vi "Test Shift Registers Loop 1.vi"() -> ()   [LabVIEW 2014]
panel:
  out "Array":string[](array[string])
  out "elements class name and label 2":string[](array[string])
  out "elements class name and label":string[](array[string])
  in  "vi path":path=path "C:/Users/lubo/Documents/LabView/LabVIEW-Universal-Transcriptor/Test/Examples For Parsing/Example System Functions.vi"
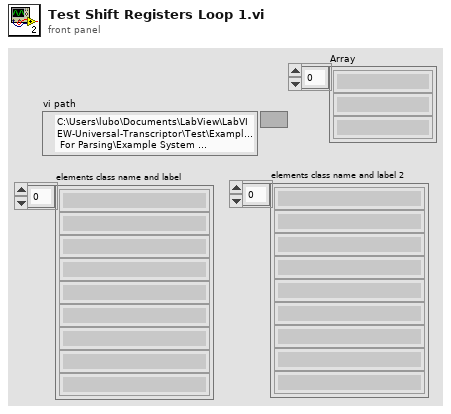
[diagram p1: front panel]
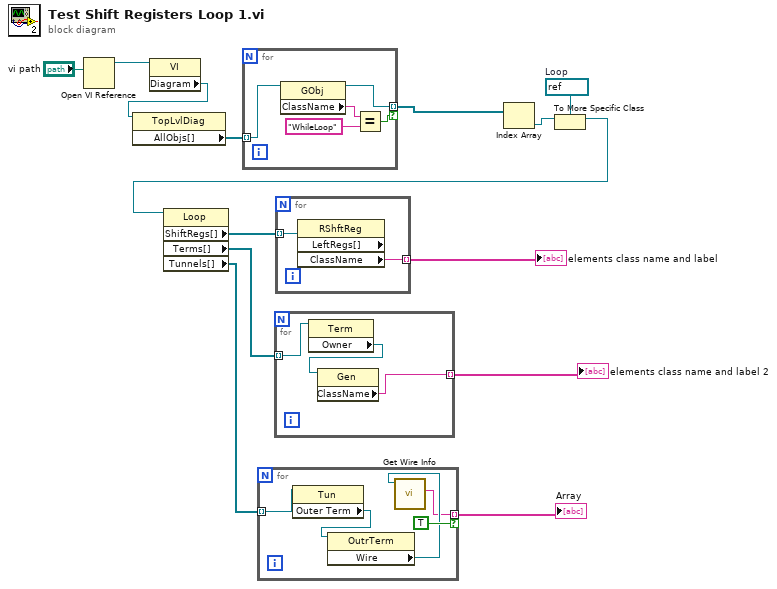
[diagram p0: block diagram]
diagram:
  w8 = refnum<vi> refnum  # Loop
  n1 = Open VI Reference(vi path="vi path") -> (vi reference=w13:refnum<vi>)  [unwired: 5 in, 1 out]
  n2 = property class="VI"(reference=w13) -> ("Diagram"=w12:refnum<vi>)  [unwired: 1 in, 2 out]
  n3 = property class="TopLvlDiag"(reference=w12) -> ("AllObjs[]"=w11:refnum<vi>[])  [unwired: 1 in, 2 out]
  n4 = for {
    tunnel: w11 -> [w19] mode=indexing
    tunnel: [w17] -> w10 mode=indexing if=w18
    n5 = property class="GObj"(reference=w19) -> (reference out=w17:refnum<vi>, "ClassName"=w15:string)  [unwired: 1 in, 1 out]
    n6 = Equal?(x=w15, y="WhileLoop") -> (x = y?=w18:bool)
  }
  n7 = Index Array(array=w10) -> (element=w9:refnum<vi>)  [unwired: 1 in]
  n8 = To More Specific Class(target class=w8, reference=w9) -> (specific class reference=w7:refnum<vi>)  [unwired: 1 in, 1 out]
  n9 = property class="Loop"(reference=w7) -> ("ShiftRegs[]"=w6:refnum<vi>[], "Terms[]"=w4:refnum<vi>[], "Tunnels[]"=w2:refnum<vi>[])  [unwired: 1 in, 2 out]
  n10 = for {
    tunnel: w2 -> [w24] mode=indexing
    tunnel: [w20] -> w1 mode=indexing if=TRUE
    n11 = property class="Tun"(reference=w24) -> ("Outer Term"=w22:refnum<vi>)  [unwired: 1 in, 2 out]
    n12 = property class="OutrTerm"(reference=w22) -> ("Wire"=w21:refnum<vi>)  [unwired: 1 in, 2 out]
    n13 = call "Get Wire Info.vi"("Wire"=w21) -> ("wire datatype"=w20:string)  [unwired: 9 in, 1 out]
  }
  "Array" <- w1
  n14 = for {
    tunnel: w4 -> [w27] mode=indexing
    tunnel: [w25] -> w3 mode=indexing
    n15 = property class="Term"(reference=w27) -> ("Owner"=w26:refnum<vi>)  [unwired: 1 in, 2 out]
    n16 = property class="Gen"(reference=w26) -> ("ClassName"=w25:string)  [unwired: 1 in, 2 out]
  }
  "elements class name and label 2" <- w3
  n17 = for {
    tunnel: w6 -> [w29] mode=indexing
    tunnel: [w28] -> w5 mode=indexing
    n18 = property class="RShftReg" props=["LeftRegs[]", "ClassName"](reference=w29) -> ("ClassName"=w28:string)  [unwired: 1 in, 3 out]
  }
  "elements class name and label" <- w5
